vi "PopUp Theme Global.vi"() -> ()   [LabVIEW 2021, in "Pop-Up.lvlib" / "Popup.lvclass"]
doc: "global variable that internally tracks the loaded theme object so that it can be updated or grabbed on the fly more easily"
uses:
  Popup.lvclass
  Theme/Theme.lvclass
panel:
  in  "temp?":bool
  in  "Theme set?":bool
  in  "Theme.lvclass":refnum<class "Theme.lvclass">
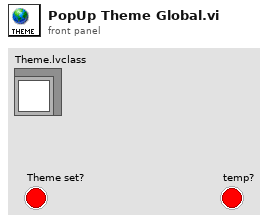
[diagram p1: front panel]
diagram:
